vi "observacao.vi"() -> ()   [LabVIEW 2018, in "Shared_160.lvlib"] (continued)
                n3095 = global read "Global_Telescopio.vi" "Precessed RA"() -> (w4054:dbl)
                n3096 = global read "Global_Telescopio.vi" "CalDEC Local"() -> (w4056:dbl)
                n3097 = global read "Global_Telescopio.vi" "Calagem AH"() -> (w4057:dbl)
                n3098 = global read "Global_Telescopio.vi" "Sideral Time"() -> (w4043:dbl)
                n3099 = global read "Global_Telescopio.vi" "CalAH Local"() -> (w4050:dbl)
                n3100 = global read "Global_Telescopio.vi" "PosDEC"() -> (w4044:dbl)
                n3101 = global read "Global_Telescopio.vi" "PosAH"() -> (w4042:dbl)
                n3102 = Subtract(x=w4052, y=w4050) -> (x-y=w4049:dbl)
                n3103 = Add(x=w4051, y=w4056) -> (x+y=w4047:dbl)
                n3104 = Subtract(x=w4043, y=w4042) -> (x-y=w4045:dbl)
                n3105 = Subtract(x=w4049, y=w4057) -> (x-y=w4048:dbl)
                n3106 = Add(x=w4047, y=w4055) -> (x+y=w4046:dbl)
                n3107 = call "rad_hms.vi"("TRUE=HORA\nFALSE=GRAU"=w4027, "Radiano"=w4054) -> ("Hora/Graus Texto Decimal"=w4030:string)  [unwired: 3 in]
                n3108 = call "rad_hms.vi"("TRUE=HORA\nFALSE=GRAU"=w4026, "Radiano"=w4053) -> ("Hora/Graus Texto Decimal"=w4031:string)  [unwired: 3 in]
                n3109 = call "rad_hms.vi"("TRUE=HORA\nFALSE=GRAU"=w4027, "Radiano"=w4052) -> ("Hora/Graus Texto Decimal"=w4032:string)  [unwired: 3 in]
                n3110 = call "rad_hms.vi"("TRUE=HORA\nFALSE=GRAU"=w4026, "Radiano"=w4051) -> ("Hora/Graus Texto Decimal"=w4033:string)  [unwired: 3 in]
                n3111 = call "rad_hms.vi"("TRUE=HORA\nFALSE=GRAU"=w4027, "Radiano"=w4049) -> ("Hora/Graus Texto Decimal"=w4034:string)  [unwired: 3 in]
                n3112 = call "rad_hms.vi"("TRUE=HORA\nFALSE=GRAU"=w4026, "Radiano"=w4047) -> ("Hora/Graus Texto Decimal"=w4035:string)  [unwired: 3 in]
                n3113 = call "rad_hms.vi"("TRUE=HORA\nFALSE=GRAU"=w4027, "Radiano"=w4048) -> ("Hora/Graus Texto Decimal"=w4036:string)  [unwired: 3 in]
                n3114 = call "rad_hms.vi"("TRUE=HORA\nFALSE=GRAU"=w4026, "Radiano"=w4046) -> ("Hora/Graus Texto Decimal"=w4037:string)  [unwired: 3 in]
                n3115 = call "rad_hms.vi"("TRUE=HORA\nFALSE=GRAU"=w4027, "Radiano"=w4045) -> ("Hora/Graus Texto Decimal"=w4038:string)  [unwired: 3 in]
                n3116 = call "rad_hms.vi"("TRUE=HORA\nFALSE=GRAU"=w4026, "Radiano"=w4044) -> ("Hora/Graus Texto Decimal"=w4039:string)  [unwired: 3 in]
                n3117 = call "rad_hms.vi"("TRUE=HORA\nFALSE=GRAU"=w4027, "Radiano"=w4043) -> ("Hora/Graus Texto Decimal"=w4040:string)  [unwired: 3 in]
                n3118 = call "rad_hms.vi"("TRUE=HORA\nFALSE=GRAU"=w4027, "Radiano"=w4042) -> ("Hora/Graus Texto Decimal"=w4041:string)  [unwired: 3 in]
                n3119 = Concatenate Strings(w4030, w4029, w4031, w4029, w4032, w4029, w4033, w4029, w4034, w4029, w4035, w4029, w4036, w4029, w4037, w4029, w4038, w4029, w4039, w4029, w4040, w4029, w4041) -> (w4028:string)
              }
              frame #4 {
                w4079 = "\t"
                # "TU safe"
                # "MUDANÇA 30-03-2024: Apenas afeta o arquivo de LOG se e somente se o nome do objeto apontado contiver o caracter @. Neste caso o LOG é feito num arquivo separado cujo nome é formado pela data (mesma do arquivo log regular) acrescido do caracter @. O conteúdo deste novo LOG apenas difere do regular pela inclusão no início de cada registro do timestamp, do nome do objeto apontado (sem o @) e dos valores de RA e DEC, em radianos, de todas as etapas do processo de apontamento."
                # "Coordenadas da precessão, modelagem erros, calagem e lidas do encoder"
                # "Condições atmosféricas"
                # "Dados de catálogo do Objeto"
                # "Tempo e posição do telescópio"
                # "Estados das variáveis de processos"
                n3120 = global read "Global_Telescopio.vi" "NAME OBJETO"() -> (w4073:string)
                n3121 = call "Get host time.vi"() -> ("BR current time"=w4058:timestamp)  [unwired: 8 in, 3 out]
                n3122 = local read "AtmosferaStr"() -> (w4077:string)
                n3123 = global read "Global_Telescopio.vi" "Data Arq LOG"() -> (w4091:string)
                n3124 = Format Date/Time String(time format string (%c)="%c%3u" ("SOMENTE DIRETORIO"), seconds (now)=w4058) -> (date/time string=w4060:string)  [unwired: 1 in]
                n3125 = Match Pattern(string=w4073, regular expression="@" ("SOMENTE DIRETORIO")) -> (before substring=w4067:string, match substring=w4070:string, after substring=w4068:string, offset past match=w4065:i32)  [unwired: 1 in]
                n3126 = Greater Or Equal To 0?(x=w4065) -> (x >= 0?=w4064:bool)
                n3127 = Concatenate Strings("C:\\TCS\\LOG\\AP_" ("SOMENTE DIRETORIO"), w4091, w4070, ".TXT" ("SOMENTE DIRETORIO")) -> (w4069:string)
                n3128 = Concatenate Strings(w4067, w4068) -> (w4061:string)
                n3129 = Concatenate Strings(w4082, w4079, w4081, w4079, w4077, w4079, w4080, "\r\n") -> (w4063:string)
                n3130 = case shown="True" w4064 {
                  tunnel: w4063 -> [w4093 w4095]
                  tunnel: [w4093 w4099] -> w4062
                  tunnel: w4061 -> [_ w4097]
                  tunnel: w4060 -> [_ w4098]
                  tunnel: w4059 -> [_ w4096]
                  frame False {
                  }
                  frame True {
                    w4094 = "\t"
                    n3131 = Concatenate Strings(w4098, w4094, w4097, w4094, w4096, w4094, w4095) -> (w4099:string)
                  }
                }
                n3132 = String To Path(string=w4069) -> (path=w4090:path)
                n3133 = call <vilib>:"Open_Create_Replace File.vi"("function (open:0)"=T9."open or create", "file path"=w4090) -> ("error out"=w4087:errorcluster, "refnum"=w4088:refnum<file>)  [unwired: 6 in, 2 out]
                n3134 = Set File Position(refnum=w4088, from (0:start)=enum16{"start", "end", "current"}."end" ("pos mode (0:2)"), error in=w4087) -> (refnum out=w4076:refnum<file>, error out=w4075:errorcluster)  [unwired: 1 in]
                n3135 = Write to Binary File(file (use dialog)=w4076, data=w4062, error in=w4075, 5:FALSE ("prepend array or string size? (T)")) -> (refnum out=w4084:refnum<file>, error out=w4085:errorcluster)  [unwired: 2 in, 1 out]
                n3136 = Close File(refnum=w4084, error in=w4085) -> (error out=w4083:errorcluster)  [unwired: 1 out]
                n3137 = call <vilib>:"Simple Error Handler.vi"("error in (no error)"=w4083) -> ()  [unwired: 4 in, 5 out]
              }
            }
          }
        }
        n3138 = case shown="False" w3920 {
          frame False {
            w3936 = u16 3 items=["Alarme", "Atencao", "Erro", "Ocupado", "Protecao", "Embreagem", "Tracking", "Var. Track", "Rápido", "Ligeiro", "Médio", "Lento", "Em movimento", ""] ("NomeStatus")
            n3139 = call "Bit Status AH.vi"("NomeStatus"=w3936) -> ("StatBit"=w3935:bool)
            n3140 = case shown="True" "MOUNT" {
              tunnel: w3935 -> [w3938 w3947]
              frame False {
                n3141 = local read "LED MOUNT"() -> (w3939:bool)
                n3142 = Not(x=w3938) -> (.not. x?=w3941:bool)
                n3143 = And(x=w3941, y=w3939) -> (x .and. y?=w3940:bool)
                n3144 = case shown="True" w3940 {
                  frame False {
                  }
                  frame True {
                    w3943 = FALSE
                    w3944 = u16 1 items=["ZERO", "AH", "DEC", "TUBO", "CUP"] ("Controlador")
                    n3145 = call "Monta Comando.vi"("Comando"="DESLIGAR", "Dispositivo"="SIDERAL" ("Comando"), "Controlador"=w3944) -> ()  [unwired: 2 in, 5 out]
                    n3146 = local write "LED MOUNT"(w3943) -> ()
                    n3147 = global write "Global_Telescopio.vi" "ObjCentrado"(w3943) -> ()
                    n3148 = property on="Calagem" class="Bool"("Disabled"=u8 2) -> ()  [unwired: 2 in, 2 out]
                  }
                }
              }
              frame True {
                n3149 = local read "LED MOUNT"() -> (w3948:bool)
                n3150 = Or(x=w3947, y=w3948) -> (x .or. y?=w3949:bool)
                n3151 = case shown="True" w3949 {
                  frame False {
                    w3950 = u16 1 items=["ZERO", "AH", "DEC", "TUBO", "CUP"] ("Controlador")
                    n3152 = call "Monta Comando.vi"("Comando"="LIGAR", "Dispositivo"="SIDERAL" ("Comando"), "Controlador"=w3950) -> ()  [unwired: 2 in, 5 out]
                    "LED MOUNT" <- TRUE
                  }
                  frame True {
                  }
                }
              }
            }
          }
          frame True {
            n3153 = local write "LED MOUNT"(FALSE) -> ()
          }
        }
      }
      frame #4 {
        # "VLC"
        # "NO_VISION 2025may"
        # "As abas de Imagens All Sky, Finder, Telescope e Image 3 foram criadas para mostrar imagens capturadas por câmeras conectadas à\nplaca grabber Angelo RTV, desativada há muito tempo. Esse recurso ainda não tinha sido removido do código do TCSPD para\nmanter exemplos de código que lida com imagens, mas finalmente removido na versão 1.0.21."
        # "ABAS DE IMAGENS"
        n3154 = case shown="\"All Sky\"" T1."Test Only" ("Tab Control") {
          frame "Image 1", Default {
          }
          frame "All Sky" {
          }
          frame "Finder" {
          }
          frame "Telescope" {
          }
          frame "Image 3" {
          }
          frame "Test Only" {
          }
        }
        n3155 = global read "Global_Telescopio.vi" "Caminho camera"() -> (w4105:string)
        n3156 = global read "Global_Telescopio.vi" "stop"() -> (w4106:bool)
        n3157 = call "Greatek.vi"("error in (no error)"="error in (no error)", "Boolean"=w4106, "name or relative path"=w4105, ".NET Refnum in"="PictureBox") -> ()  [unwired: 7 in, 1 out]
      }
      frame #5 {
        w4109 = u16 15 items=["Alarme", "Atencao", "Erro", "Ocupado", "Plataforma", "LCB", "Trapeira", "Paravento", "DomoRap", "DomoCW", "DomoCCW", "TBD", "Em movimento", "TrapRUN", "TrapFCH", "TrapABT"] ("NomeStatus")
        w4120 = u16 4 items=["Alarme", "Atencao", "Erro", "Ocupado", "Plataforma", "LCB", "Trapeira", "Paravento", "DomoRap", "DomoCW", "DomoCCW", "TBD", "Em movimento", "TrapRUN", "TrapFCH", "TrapABT"] ("NomeStatus")
        w4122 = u16 15 items=["Alarme", "Atencao", "Erro", "Ocupado", "Plataforma", "LCB", "Trapeira", "Paravento", "DomoRap", "DomoCW", "DomoCCW", "TBD", "Em movimento", "TrapRUN", "TrapFCH", "TrapABT"] ("NomeStatus")
        w4137 = u16 3 items=["Alarme", "Atencao", "Erro", "Ocupado", "TBD", "LCB", "Trapeira", "Paravento", "DomoRap", "DomoCW", "DomoCCW", "TBD", "Em movimento", "TBD"] ("NomeStatus")
        # "20250912"
        # "ZeroMQ"
        # "JANELA DE STATUS"
        n3158 = local read "RA on Target"() -> (w4133:bool)
        n3159 = local read "DEC on Target"() -> (w4132:bool)
        n3160 = local read "Led Chave Dome"() -> (w4129:bool)
        n3161 = local read "Dome on Target"() -> (w4131:bool)
        n3162 = local read "LED GUIDER"() -> (w4128:bool)
        n3163 = local read "MOUNT"() -> (w4130:bool)
        n3164 = local read "Mount Gross Movement"() -> (w4127:bool)
        n3165 = local read "Mount Fine Movement"() -> (w4126:bool)
        n3166 = local read "ObjCentrado"() -> (w4125:bool)
        n3167 = local read "LED VAR TRACKING"() -> (w4124:bool)
        n3168 = local read "StatDome"() -> (w4123:string)
        n3169 = local read "OpenShutterPassword"() -> (w4116:string)
        n3170 = global read "Global_Telescopio.vi" "Senha LEAF"() -> (w4111:string)
        n3171 = call "Bit Status CUP.vi"("NomeStatus"=w4109) -> ("StatBit"=w4110:bool)
        n3172 = local read "ChkDomeEnable"() -> (w4148:bool)
        n3173 = local read "Flag Stop"() -> (w4143:bool)
        n3174 = global write "Global_Telescopio.vi" "PUB RA on Target"(w4133) -> ()
        n3175 = global write "Global_Telescopio.vi" "PUB DEC on Target"(w4132) -> ()
        n3176 = global write "Global_Telescopio.vi" "PUB Dome"(w4129) -> ()
        n3177 = global write "Global_Telescopio.vi" "PUB Dome on Target"(w4131) -> ()
        n3178 = global write "Global_Telescopio.vi" "PUB GUIDER"(w4128) -> ()
        n3179 = global write "Global_Telescopio.vi" "PUB MOUNT"(w4130) -> ()
        n3180 = global write "Global_Telescopio.vi" "PUB Mount Gross Movement"(w4127) -> ()
        n3181 = global write "Global_Telescopio.vi" "PUB Mount Fine Movement"(w4126) -> ()
        n3182 = global write "Global_Telescopio.vi" "PUB ObjCentrado"(w4125) -> ()
        n3183 = global write "Global_Telescopio.vi" "PUB VAR TRACKING"(w4124) -> ()
        n3184 = global write "Global_Telescopio.vi" "PUB StatDome"(w4123) -> ()
        n3185 = global write "Global_Telescopio.vi" "PUB SHUTTER"(w4110) -> ()
        n3186 = call "Bit Status CUP.vi"("NomeStatus"=w4120) -> ("StatBit"=w4113:bool)
        n3187 = Match Pattern(string=w4116, regular expression=w4111) -> (offset past match=w4115:i32)  [unwired: 1 in, 3 out]
        n3188 = call "Bit Status CUP.vi"("NomeStatus"=w4122) -> ("StatBit"=→"Shutter opened":bool)
        n3189 = case shown="True" w4148 {
          tunnel: [TRUE ("AUX LAMPADA") w4301] -> w4147
          frame False {
          }
          frame True {
            w4307 = u16 3 items=["Alarme", "Atencao", "Erro", "Ocupado", "TBD", "LCB", "Trapeira", "Paravento", "DomoRap", "DomoCW", "DomoCCW", "TBD", "Em movimento", "TBD"] ("NomeStatus")
            n3190 = local read "Dome on Target"() -> (w4304:bool)
            n3191 = local read "statCUP"() -> (w4306:i32)
            n3192 = call "Bit Status CUP.vi"("NomeStatus"=w4307) -> ("StatBit"=w4303:bool)
            n3193 = Equal To 0?(x=w4306) -> (x = 0?=w4305:bool)
            n3194 = Not(x=w4303) -> (.not. x?=w4302:bool)
            n3195 = Compound Arithmetic op=AND(w4305, w4304, w4302) -> (w4301:bool)
          }
        }
        n3196 = case shown="True" w4143 {
          tunnel: [FALSE w4294] -> w4142
          frame False {
          }
          frame True {
            w4298 = u16 3 items=["Alarme", "Atencao", "Erro", "Ocupado", "TBD", "LCB", "Trapeira", "Paravento", "DomoRap", "DomoCW", "DomoCCW", "TBD", "Em movimento", "TBD"] ("NomeStatus")
            n3197 = local read "statCUP"() -> (w4297:i32)
            n3198 = call "Bit Status CUP.vi"("NomeStatus"=w4298) -> ("StatBit"=w4299:bool)
            n3199 = Equal To 0?(x=w4297) -> (x = 0?=w4296:bool)
            n3200 = Not(x=w4299) -> (.not. x?=w4295:bool)
            n3201 = Compound Arithmetic op=AND(w4296, w4295) -> (w4294:bool)
          }
        }
        n3202 = Greater Or Equal To 0?(x=w4115) -> (x >= 0?=w4114:bool)
        n3203 = Not(x=w4113) -> (.not. x?=w4107:bool)
        "Plataform" <- w4107
        n3204 = Or(x=w4113, y=w4114) -> (x .or. y?=w4112:bool)
        n3205 = local read "Flag de erro p/ apagar lampada"() -> (w4138:bool)
        n3206 = property on="Plataform" class="Bool (strict)"("Blinking"=w4107) -> ()  [unwired: 2 in, 2 out]
        n3207 = global write "Global_Telescopio.vi" "PUB AlarmePlataforma"(w4107) -> ()
        n3208 = Select(t=T5."Enabled" ("Disabled"), s=w4112, f=T5."Disabled" ("Disabled")) -> (s? t:f=w4117:T5)
        n3209 = call "Bit Status CUP.vi"("NomeStatus"=w4137) -> ("StatBit"=w4136:bool)
        n3210 = local read "DEC on Target"() -> (w4149:bool)
        n3211 = local read "RA on Target"() -> (w4150:bool)
        n3212 = property on="BtTargetPoint" class="Bool"("DisabledEnum"=w4117) -> ()  [unwired: 2 in, 2 out]
        n3213 = property on="FLAT-FIELD" class="Bool (strict)"("DisabledEnum"=w4117) -> ()  [unwired: 2 in, 2 out]
        n3214 = property on="ECASS" class="Bool (strict)"("DisabledEnum"=w4117) -> ()  [unwired: 2 in, 2 out]
        n3215 = property on="BtUtilZenith" class="Bool (strict)"("DisabledEnum"=w4117) -> ()  [unwired: 2 in, 2 out]
        n3216 = local read "Apontou"() -> (w4108:bool)
        n3217 = local read "BtUtilZenith"() -> (w4162:bool)
        n3218 = local read "BtUtilPark"() -> (w4161:bool)
        n3219 = local read "BtUtilZenith"() -> (w4160:bool)
        n3220 = local read "ECASS"() -> (w4159:bool)
        n3221 = local read "FLAT-FIELD"() -> (w4158:bool)
        n3222 = Not(x=w4136) -> (.not. x?=w4135:bool)
        n3223 = Compound Arithmetic op=OR(w4108, w4162, w4161, w4160, w4159, w4158) -> (w4155:bool)
        n3224 = Compound Arithmetic op=AND(w4138, w4135) -> (w4134:bool)
        n3225 = Compound Arithmetic op=AND(w4150, w4149, w4147) -> (w4146:bool)
        n3226 = And(x=w4146, y="AUX LAMPADA") -> (x .and. y?=w4144:bool)
        n3227 = Or(x=w4144, y=w4142) -> (x .or. y?=w4139:bool)
        n3228 = Or(x=w4139, y=w4134) -> (x .or. y?=w4140:bool)
        n3229 = And(x=w4155, y="AUX ABA") -> (x .and. y?=w4157:bool)
        n3230 = Not(x=w4150) -> (.not. x?=w4151:bool)
        n3231 = Not(x=w4149) -> (.not. x?=w4153:bool)
        n3232 = Not(x=w4147) -> (.not. x?=w4152:bool)
        n3233 = case shown="True" w4140 {
          selector: w4140 -> [_ w4312]
          frame False {
          }
          frame True {
            w4309 = u16 4 items=["ZERO", "AH", "DEC", "TUBO", "CUP"] ("Controlador")
            n3234 = Not(x=w4312) -> (.not. x?=w4308:bool)
            n3235 = local write "AUX LAMPADA"(w4308) -> ()
            n3236 = local write "Flag Stop"(w4308) -> ()
            n3237 = local write "Flag de erro p/ apagar lampada"(w4308) -> ()
            n3238 = local write "Tab Control"(T1."Test Only" ("Tab Control")) -> ()
            n3239 = call "Monta Comando.vi"("Comando"="DESLIGAR", "Dispositivo"="LAMP_CAM", "Controlador"=w4309) -> ()  [unwired: 2 in, 5 out]
          }
        }
        n3240 = case shown="True" w4157 {
          selector: w4157 -> [_ w4320]
          frame False {
          }
          frame True {
            # "Liga a câmera de monitoramento"
            # "Ligar a lâmpada pra a câmera"
            n3241 = Not(x=w4320) -> (.not. x?=w4319:bool)
            n3242 = local write "AUX LAMPADA"(TRUE ("AUX LAMPADA")) -> ()
            n3243 = local write "Tab Control"(T1."Image 1" ("Tab Control")) -> ()
            n3244 = local write "AUX ABA"(w4319) -> ()
            n3245 = local write "Apontou"(w4319) -> ()
            n3246 = call <vilib>:"System Exec.vi"("command line"="C:\\TCS\\ARQUIVOS\\camera.xspf") -> ()  [unwired: 7 in, 4 out]
          }
        }
        n3247 = case shown="False" w4155 {
          selector: w4155 -> [w4315 _]
          frame False {
            n3248 = Not(x=w4315) -> (.not. x?=w4316:bool)
            n3249 = local write "AUX ABA"(w4316) -> ()
          }
          frame True {
          }
        }
        n3250 = Compound Arithmetic op=OR(w4151, w4153, w4152) -> (w4154:bool)
        n3251 = case shown="True" w4154 {
          selector: w4154 -> [_ w4314]
          frame False {
          }
          frame True {
            n3252 = local write "AUX LAMPADA"(w4314) -> ()
          }
        }
        n3253 = global read "Global_Telescopio.vi" "Enable ventilador"() -> (w4141:bool)
        n3254 = Tick Count (ms)() -> (millisecond timer value=w4165:u32)
        n3255 = case shown="True" w4141 {
          frame False {
          }
          frame True {
            w4171 = u16 3 items=["Alarme", "Atencao", "Erro", "Ocupado", "TBD", "LCB", "Trapeira", "Paravento", "DomoRap", "DomoCW", "DomoCCW", "TBD", "Em movimento", "TBD"] ("NomeStatus")
            n3256 = global read "Global_Telescopio.vi" "Hora vent inicial"() -> (w4168:string)
            n3257 = global read "Global_Telescopio.vi" "Hora vent final"() -> (w4167:string)
            n3258 = call "Bit Status TUBO.vi"("NomeStatus"=w4171) -> ("StatBit"=w4170:bool)
            n3259 = call "Comp-HorarioSeg.vi"("Lower limit"=w4168, "Upper limit"=w4167) -> ("In Range?"=w4166:bool)
            n3260 = Not(x=w4170) -> (.not. x?=w4169:bool)
            n3261 = case shown="\"erro_ligar\"" "xxz" {
              tunnel: [w4174 w4199 w4224 w4228 w4241 w4247 w4260] -> w4172
              tunnel: w4166 -> [_ _ w4223 _ w4243 _ w4261]
              tunnel: w4169 -> [w4175 w4200 _ w4227 w4242 w4246 _]
              frame "erro_ligar" {
                n3262 = case shown="True" w4175 {
                  tunnel: ["erro_ligar" w4178] -> w4174
                  frame False {
                  }
                  frame True {
                    w4187 = u16 3 items=["ZERO", "AH", "DEC", "TUBO", "CUP"] ("Controlador")
                    # "super erro"
                    n3263 = call "Monta Comando.vi"("Comando"="LIGAR", "Dispositivo"="VENTILADOR", "Controlador"=w4187) -> ("Resposta"=w4190:string, "cmdT"=→"cmdT":string)  [unwired: 2 in, 3 out]
                    n3264 = String Subset(string=w4190, length (rest)=3 ("length (rest)")) -> (substring=w4184:string)  [unwired: 1 in]
                    n3265 = Equal?(x=w4184, y="ACK") -> (x = y?=w4180:bool)
                    n3266 = case shown="False" w4180 {
                      tunnel: [w4191 FALSE] -> w4181
                      tunnel: "erro_ligar" -> [w4192 _]
                      tunnel: [w4192 "espera_desligar"] -> w4179
                      frame False {
                        n3267 = Increment(x="erro lig") -> (x+1=w4193:i32)
                        n3268 = local write "erro lig"(w4193) -> ()
                        n3269 = Greater Or Equal?(x=w4193, y=3) -> (x >= y?=w4191:bool)
                        n3270 = case shown="True" w4191 {
                          frame False {
                          }
                          frame True {
                            w4196 = "Erro de acionamento do ventilador do tubo" ("SYSTEM MESSAGES")
                            n3271 = call "Monta_Mensagem.vi"("Mensagem"=w4196) -> ()  [unwired: 2 in]
                            n3272 = call "Salva_systems_messages.vi"("Mensagem"=w4196) -> ()  [unwired: 5 in]
                          }
                        }
                      }
                      frame True {
                      }
                    }
                    n3273 = Select(t="espera_desligar", s=w4181, f=w4179) -> (s? t:f=w4178:string)
                  }
                }
              }
              frame "erro_desligar" {
                n3274 = case shown="True" w4200 {
                  tunnel: ["erro_desligar" w4202] -> w4199
                  frame False {
                  }
                  frame True {
                    w4212 = u16 3 items=["ZERO", "AH", "DEC", "TUBO", "CUP"] ("Controlador")
                    # "super erro"
                    n3275 = call "Monta Comando.vi"("Comando"="DESLIGAR", "Dispositivo"="VENTILADOR", "Controlador"=w4212) -> ("Resposta"=w4210:string)  [unwired: 2 in, 4 out]
                    n3276 = String Subset(string=w4210, length (rest)=3 ("length (rest)")) -> (substring=w4208:string)  [unwired: 1 in]
                    n3277 = Equal?(x=w4208, y="ACK") -> (x = y?=w4207:bool)
                    n3278 = case shown="False" w4207 {
                      tunnel: [w4215 FALSE] -> w4206
                      tunnel: "erro_desligar" -> [w4216 _]
                      tunnel: [w4216 "aguardando _ligar"] -> w4204
                      frame False {
                        n3279 = Increment(x="erro des") -> (x+1=w4218:i32)
                        n3280 = local write "erro des"(w4218) -> ()
                        n3281 = Greater Or Equal?(x=w4218, y=3) -> (x >= y?=w4215:bool)
                        n3282 = case shown="True" w4215 {
                          frame False {
                          }
                          frame True {
                            w4220 = "Erro de acionamento do ventilador do tubo" ("SYSTEM MESSAGES")
                            n3283 = call "Monta_Mensagem.vi"("Mensagem"=w4220) -> ()  [unwired: 2 in]
                            n3284 = call "Salva_systems_messages.vi"("Mensagem"=w4220) -> ()  [unwired: 5 in]
                          }
                        }
                      }
                      frame True {
                      }
                    }
                    n3285 = Select(t="aguardando _ligar", s=w4206, f=w4204) -> (s? t:f=w4202:string)
                  }
                }
              }
              frame "inicio", Default {
                n3286 = Select(t="ligar", s=w4223, f="desligar") -> (s? t:f=w4224:string)
              }
              frame "ligar" {
                n3287 = case shown="False" w4227 {
                  tunnel: ["ligar" w4231] -> w4228
                  frame False {
                  }
                  frame True {
                    w4238 = u16 3 items=["ZERO", "AH", "DEC", "TUBO", "CUP"] ("Controlador")
                    n3288 = call "Monta Comando.vi"("Comando"="LIGAR", "Dispositivo"="VENTILADOR", "Controlador"=w4238) -> ("Resposta"=w4236:string)  [unwired: 2 in, 4 out]
                    n3289 = String Subset(string=w4236, length (rest)=3 ("length (rest)")) -> (substring=w4234:string)  [unwired: 1 in]
                    n3290 = Equal?(x=w4234, y="ACK") -> (x = y?=w4230:bool)
                    n3291 = Select(t="espera_desligar", s=w4230, f="erro_ligar") -> (s? t:f=w4231:string)
                  }
                }
              }
              frame "espera_desligar" {
                n3292 = case shown="False" w4243 {
                  tunnel: w4242 -> [_ _]
                  tunnel: ["desligar" "espera_desligar"] -> w4241
                  frame False {
                    # "Já ligou mas saiu da faixa e deve desligar"
                  }
                  frame True {
                    # "Já ligou mas está na faixa"
                  }
                }
              }
              frame "desligar" {
                n3293 = case shown="True" w4246 {
                  tunnel: ["desligar" w4249] -> w4247
                  frame False {
                  }
                  frame True {
                    w4257 = u16 3 items=["ZERO", "AH", "DEC", "TUBO", "CUP"] ("Controlador")
                    n3294 = call "Monta Comando.vi"("Comando"="DESLIGAR", "Dispositivo"="VENTILADOR", "Controlador"=w4257) -> ("Resposta"=w4255:string)  [unwired: 2 in, 4 out]
                    n3295 = String Subset(string=w4255, length (rest)=3 ("length (rest)")) -> (substring=w4253:string)  [unwired: 1 in]
                    n3296 = Equal?(x=w4253, y="ACK") -> (x = y?=w4252:bool)
                    n3297 = Select(t="aguardando _ligar", s=w4252, f="erro_desligar") -> (s? t:f=w4249:string)
                  }
                }
              }
              frame "aguardando _ligar" {
                n3298 = case shown="True" w4261 {
                  tunnel: ["aguardando _ligar" "ligar"] -> w4260
                  frame False {
                  }
                  frame True {
                  }
                }
              }
            }
            n3299 = local write "xxz"(w4172) -> ()
          }
        }
        n3300 = stacked-sequence {
          frame #0 {
            n3301 = call "Safe Date-Time String.vi"() -> ("Safe time string"=w4264:string)  [unwired: 3 in, 1 out]
            n3302 = In Range and Coerce(upper limit="16:00:01", x=w4264, lower limit="15:59:59" ("upper limit")) -> (In Range?=w4266:bool)  [unwired: 1 out]
            n3303 = In Range and Coerce(upper limit="17:45:01", x=w4264, lower limit="17:44:59" ("upper limit")) -> (In Range?=w4265:bool)  [unwired: 1 out]
            n3304 = case shown="True" w4265 {
              selector: w4265 -> [_ w4271]
              frame False {
              }
              frame True {
                "Flag desligar" <- w4271
              }
            }
            n3305 = case shown="True" w4266 {
              selector: w4266 -> [_ w4272]
              frame False {
              }
              frame True {
                "Flag ligar" <- w4272
              }
            }
          }
          frame #1 {
            n3306 = local read "Flag ligar"() -> (w4274:bool)
            n3307 = local read "Flag desligar"() -> (w4273:bool)
            n3308 = Or(x=w4274, y=w4273) -> (x .or. y?=w4275:bool)
            n3309 = case shown="True" w4275 {
              tunnel: w4274 -> [_ w4276]
              tunnel: w4273 -> [_ w4278]
              frame False {
              }
              frame True {
                w4282 = u16 3 items=["Alarme", "Atencao", "Erro", "Ocupado", "TBD", "LCB", "Trapeira", "Paravento", "DomoRap", "DomoCW", "DomoCCW", "TBD", "Em movimento", "TBD"] ("NomeStatus")
                n3310 = call "Bit Status TUBO.vi"("NomeStatus"=w4282) -> ("StatBit"=w4281:bool)
                n3311 = Not(x=w4281) -> (.not. x?=w4277:bool)
                n3312 = And(x=w4277, y=w4278) -> (x .and. y?=w4279:bool)
                n3313 = And(x=w4276, y=w4277) -> (x .and. y?=w4280:bool)
                n3314 = case shown="True" w4280 {
                  selector: w4280 -> [_ w4292]
                  frame False {
                  }
                  frame True {
                    w4290 = u16 3 items=["ZERO", "AH", "DEC", "TUBO", "CUP"] ("Controlador")
                    n3315 = Not(x=w4292) -> (.not. x?=w4291:bool)
                    n3316 = local write "Flag ligar"(w4291) -> ()
                    n3317 = call "Monta Comando.vi"("Comando"="LIGAR", "Dispositivo"="VENTILADOR", "Controlador"=w4290) -> ()  [unwired: 2 in, 5 out]
                  }
                }
                n3318 = case shown="True" w4279 {
                  selector: w4279 -> [_ w4287]
                  frame False {
                  }
                  frame True {
                    w4283 = u16 3 items=["ZERO", "AH", "DEC", "TUBO", "CUP"] ("Controlador")
                    n3319 = Not(x=w4287) -> (.not. x?=w4286:bool)
                    n3320 = local write "Flag desligar"(w4286) -> ()
                    n3321 = call "Monta Comando.vi"("Comando"="DESLIGAR", "Dispositivo"="VENTILADOR", "Controlador"=w4283) -> ()  [unwired: 2 in, 5 out]
                  }
                }
              }
            }
          }
        }
        n3322 = Subtract(x=w4165, y=w4164) -> (x-y=→"dt":u32)
      }
    }
    n3323 = Wait Until Next ms Multiple(millisecond multiple=u32 100) -> ()  [unwired: 1 out]
    n3324 = global read "Global_Telescopio.vi" "stop"() -> (w91:bool)
    n3325 = Or(x=w91, y="sair") -> (x .or. y?=w92:bool)
  }
  n3326 = flat-sequence {
    tunnel: w1 -> [_]
    frame #0 {
      # "Destói filas para comunicação com os controladores"
      # "Comando EXIT P/ O VI QBRIDGE"
      # "Libera as filas do focalizador"
      n3327 = global read "Global_Telescopio.vi" "queueSUB"() -> (w4333:refnum<queue>)
      n3328 = global read "Global_Telescopio.vi" "queuePUSH"() -> (w4332:refnum<queue>)
      n3329 = global read "Global_Telescopio.vi" "queueRespAH"() -> (w4328:refnum<queue>)
      n3330 = global read "Global_Telescopio.vi" "queueCmdAH"() -> (w4329:refnum<queue>)
      n3331 = global read "Global_Telescopio.vi" "queueRespDEC"() -> (w4327:refnum<queue>)
      n3332 = global read "Global_Telescopio.vi" "queueCmdDEC"() -> (w4326:refnum<queue>)
      n3333 = global read "Global_Telescopio.vi" "queueRespTUBO"() -> (w4324:refnum<queue>)
      n3334 = global read "Global_Telescopio.vi" "queueCmdTUBO"() -> (w4325:refnum<queue>)
      n3335 = global read "Global_Telescopio.vi" "queueRespCUP"() -> (w4322:refnum<queue>)
      n3336 = global read "Global_Telescopio.vi" "queueCmdCUP"() -> (w4323:refnum<queue>)
      n3337 = Enqueue Element(queue=w4332, element="AbortBridge") -> (queue out=w4331:refnum<queue>)  [unwired: 2 in, 2 out]
      n3338 = Release Queue(queue=w4328) -> ()  [unwired: 2 in, 3 out]
      n3339 = Release Queue(queue=w4329) -> ()  [unwired: 2 in, 3 out]
      n3340 = Release Queue(queue=w4327) -> ()  [unwired: 2 in, 3 out]
      n3341 = Release Queue(queue=w4326) -> ()  [unwired: 2 in, 3 out]
      n3342 = Release Queue(queue=w4324) -> ()  [unwired: 2 in, 3 out]
      n3343 = Release Queue(queue=w4325) -> ()  [unwired: 2 in, 3 out]
      n3344 = Release Queue(queue=w4322) -> ()  [unwired: 2 in, 3 out]
      n3345 = Release Queue(queue=w4323) -> ()  [unwired: 2 in, 3 out]
      n3346 = Release Queue(queue=w4333) -> ()  [unwired: 2 in, 3 out]
      n3347 = Release Queue(queue=w4331) -> ()  [unwired: 2 in, 3 out]
    }
  }
